vi "capex chiller.vi"() -> ()   [LabVIEW 2013]
panel:
  in  "stop":bool
  out "Chiller malfunction":bool
  in  "Chiller pump speed":dbl(ring) items=["Low", "Med", "High"]
  out "Waveform Chart":dbl[](graph)
  out "Process value":dbl
  in  "Setpoint":dbl
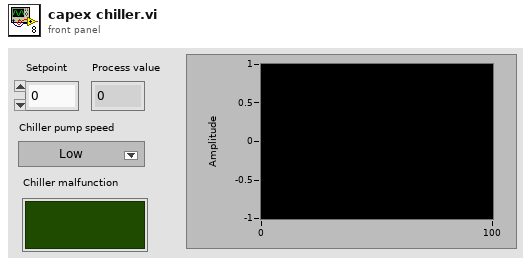
[diagram p1: front panel]
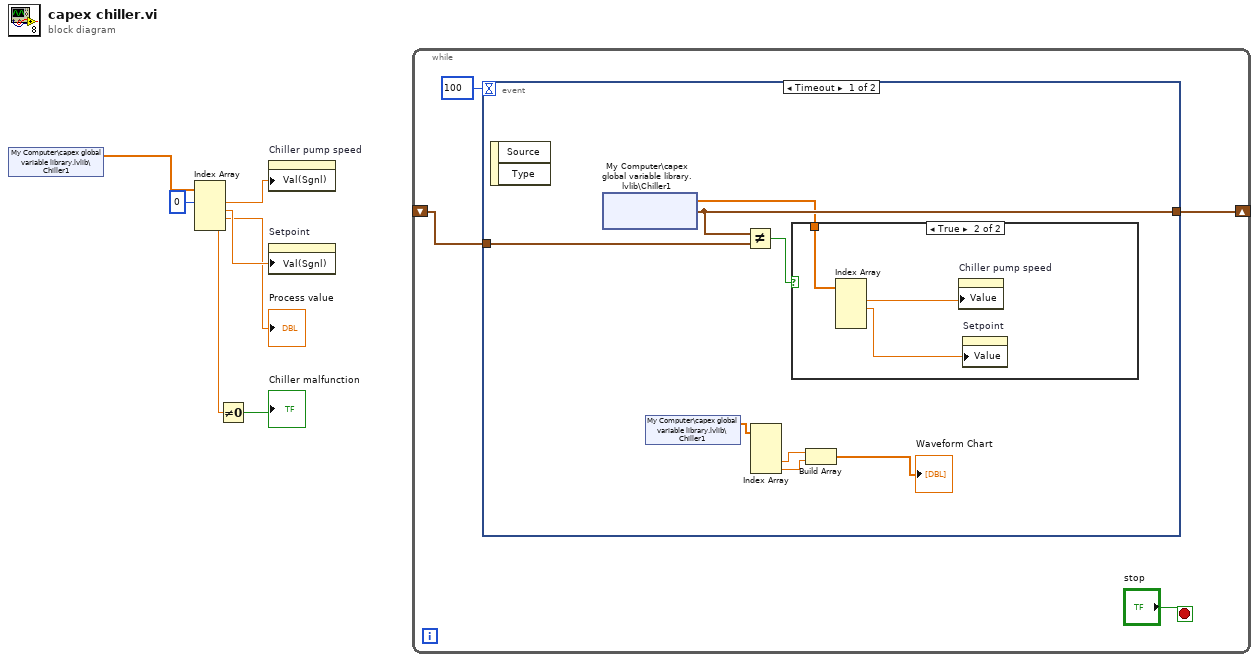
[diagram p0: block diagram]
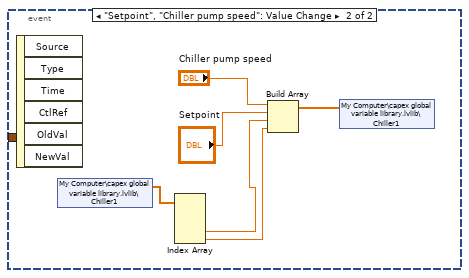
[diagram p3: hidden frame]
diagram:
  n1 = shared-variable "My Computer\\capex global variable library.lvlib\\Chiller1"() -> (w4:dbl[])  [unwired: 1 in, 1 out]
  n2 = Index Array(array=w4, index #1=0 ("index")) -> (element #1=w7:dbl, element #2=w6:dbl, element #3=→"Process value":dbl, element #4=w1:dbl)  [unwired: 3 in]
  n3 = Not Equal To 0?(x=w1) -> (x != 0?=→"Chiller malfunction":bool)
  n4 = property on="Chiller pump speed" class="Ring (strict)"("Val(Sgnl)"=w7) -> ()  [unwired: 2 in, 2 out]
  n5 = property on="Setpoint" class="DigNum (strict)"("Val(Sgnl)"=w6) -> ()  [unwired: 2 in, 2 out]
  n6 = while {
    shift-right: [w9] -> _
    shift-left: _ -> [w8]
    stop <- "stop" stop-if-true
    n7 = event shown="[0] Timeout" {
      selector: _ -> [_ _]
      dyn-events: _ -> [_ _]
      timeout: 100 -> [_ _]
      tunnel: [w17 _] -> w9
      tunnel: w8 -> [w16 _]
      event Timeout {
        n8 = event-data() -> ()  [unwired: 1 in, 2 out]
        n9 = shared-variable "My Computer\\capex global variable library.lvlib\\Chiller1"() -> (w12:dbl[], w17:timestamp)  [unwired: 1 in, 1 out]
        n10 = shared-variable "My Computer\\capex global variable library.lvlib\\Chiller1"() -> (w19:dbl[])  [unwired: 1 in, 1 out]
        n11 = Not Equal?(x=w17, y=w16) -> (x != y?=w15:bool)
        n12 = Index Array(array=w19) -> (element #3=w14:dbl, element #4=w13:dbl)  [unwired: 4 in, 2 out]
        n13 = case shown="True" w15 {
          tunnel: w12 -> [_ w22]
          frame False {
          }
          frame True {
            n14 = Index Array(array=w22) -> (element #1=w21:dbl, element #2=w20:dbl)  [unwired: 4 in, 2 out]
            n15 = property on="Chiller pump speed" class="Ring (strict)"("Value"=w21) -> ()  [unwired: 2 in, 2 out]
            n16 = property on="Setpoint" class="DigNum (strict)"("Value"=w20) -> ()  [unwired: 2 in, 2 out]
          }
        }
        n17 = Build Array(w14, w13) -> (→"Waveform Chart":dbl[])
      }
      event "Setpoint", "Chiller pump speed": Value Change {
        n18 = event-data() -> ()  [unwired: 1 in, 6 out]
        n19 = shared-variable "My Computer\\capex global variable library.lvlib\\Chiller1"() -> (w25:dbl[])  [unwired: 1 in, 1 out]
        n20 = Index Array(array=w25) -> (element #3=w24:dbl, element #4=w23:dbl)  [unwired: 4 in, 2 out]
        n21 = Build Array("Chiller pump speed", "Setpoint", w24, w23) -> (w26:dbl[])
        n22 = shared-variable "My Computer\\capex global variable library.lvlib\\Chiller1"(w26) -> ()  [unwired: 1 in, 1 out]
      }
    }
  }
